vi "buildSetTemperature.vi"(8 "error in (no error)":errorcluster, 10 "temperature[°C]":i32, 11 "PlainTextCommandBuilder in":refnum<class "PlainTextCommandBuilder.lvclass">) -> (0 "error out":errorcluster, 2 "message":string, 3 "PlainTextCommandBuilder out":refnum<class "PlainTextCommandBuilder.lvclass">)   [LabVIEW 2023, in "AbstractFactory.lvlib" / "PlainTextCommandBuilder.lvclass"]
uses:
  PlainTextCommandBuilder.lvclass
  PlainTextCommandBuilder.lvclass/PlainTextCommandBuilder.ctl
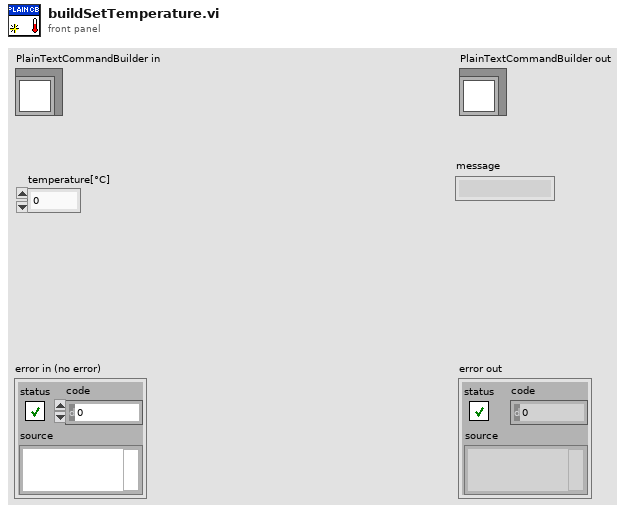
[diagram p1: front panel]
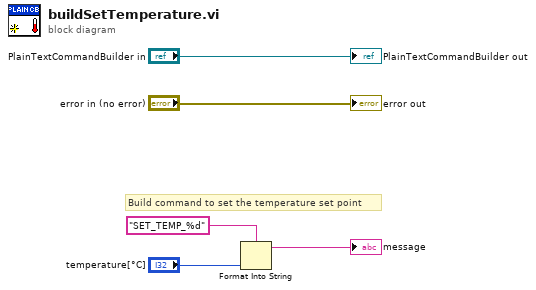
[diagram p0: block diagram]
diagram:
  # "Build command to set the temperature set point"
  n1 = Format Into String(format string="SET_TEMP_%d", "temperature[°C]") -> (resulting string=→"message":string)  [unwired: 2 in, 1 out]
  "error out" <- "error in (no error)"
  "PlainTextCommandBuilder out" <- "PlainTextCommandBuilder in"
